vi "ConvertTraceFormatElementsToItemList.vi"(11 "Trace Format Elements":T1[](array[typedef])) -> (3 "Item List":string)   [LabVIEW 2012, in "Keithley-6482.lvlib"]
uses:
  Public/Controls/TraceFormatElement.ctl
  Keithley-6482.lvlib
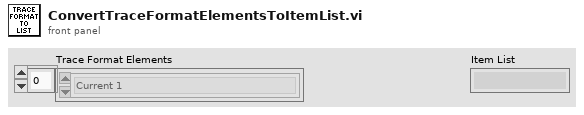
[diagram p1: front panel]
types:
  T1 = typedef "Keithley-6482.lvlib/TraceFormatElement.ctl" = enum16{"Current 1", "Current 2", "Calculate 1", "Calculate 2", "Calculate 3", "Calculate 4", "Calculate 5", "Calculate 6", "Calculate 7", "Time", "Status", "All", "Default"}
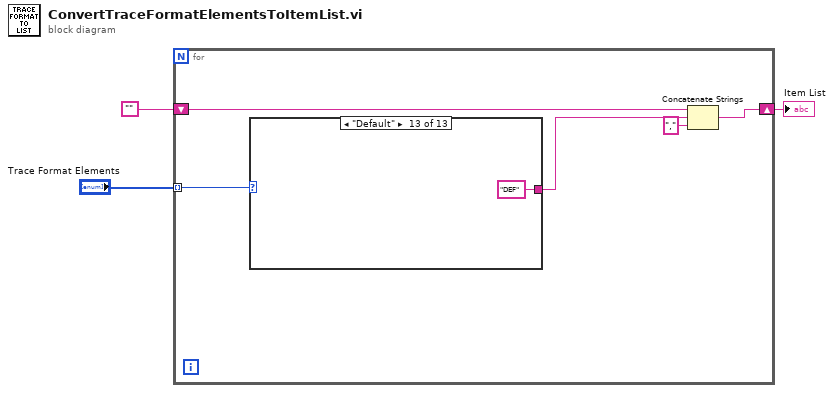
[diagram p0: block diagram]
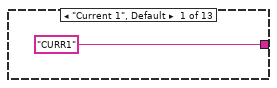
[diagram p2: hidden frame]
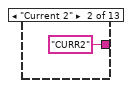
[diagram p3: hidden frame]
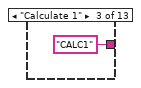
[diagram p4: hidden frame]
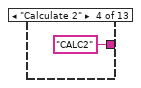
[diagram p5: hidden frame]
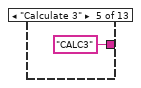
[diagram p6: hidden frame]
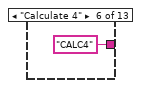
[diagram p7: hidden frame]
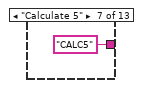
[diagram p8: hidden frame]
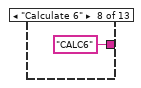
[diagram p9: hidden frame]
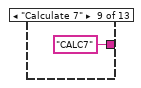
[diagram p10: hidden frame]
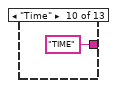
[diagram p11: hidden frame]
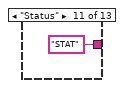
[diagram p12: hidden frame]
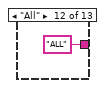
[diagram p13: hidden frame]
diagram:
  n1 = for {
    tunnel: "Trace Format Elements" -> [w6] mode=indexing
    shift-right: [w7] -> w1
    shift-left: "" -> [w8]
    n2 = case shown="\"Default\"" w6 {
      tunnel: ["CURR1" "CURR2" "CALC1" "CALC2" "CALC3" "CALC4" "CALC5" "CALC6" "CALC7" "TIME" "STAT" "ALL" "DEF"] -> w5
      frame "Current 1", Default {
      }
      frame "Current 2" {
      }
      frame "Calculate 1" {
      }
      frame "Calculate 2" {
      }
      frame "Calculate 3" {
      }
      frame "Calculate 4" {
      }
      frame "Calculate 5" {
      }
      frame "Calculate 6" {
      }
      frame "Calculate 7" {
      }
      frame "Time" {
      }
      frame "Status" {
      }
      frame "All" {
      }
      frame "Default" {
      }
    }
    n3 = Concatenate Strings(w8, w5, "," ("string")) -> (w7:string)
  }
  "Item List" <- w1
